vi "CBL Write Block.vi"(4 "TimeOut":u32, 5 "DataNum":u32, 6 "pData":string, 7 "FlashStartAddr":u32, 8 "error in (no error)":errorcluster, 9 "NodeAddr":u8, 10 "CANIndex":i32, 11 "DevIndex":i32) -> (0 "error out":errorcluster, 3 "function return":i32)   [LabVIEW 2012, in "CANBootloader.lvlib"]
doc: "int WINAPI CBL_WriteBlock(int DevIndex,int CANIndex,unsigned char NodeAddr,unsigned int FlashStartAddr,unsigned char *pData,unsigned int DataNum,unsigned int TimeOut);"
uses:
  CANBootloader.lvlib
  Ginkgo_Driver.dll
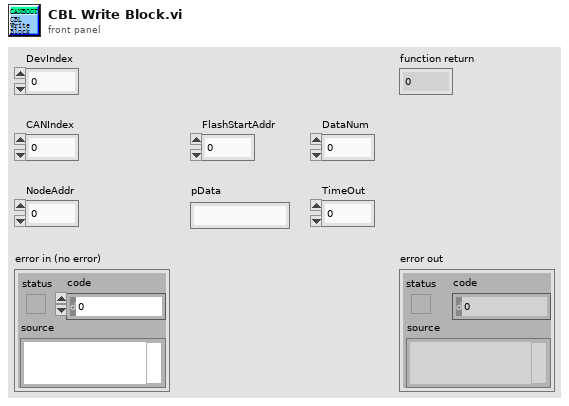
[diagram p1: front panel]
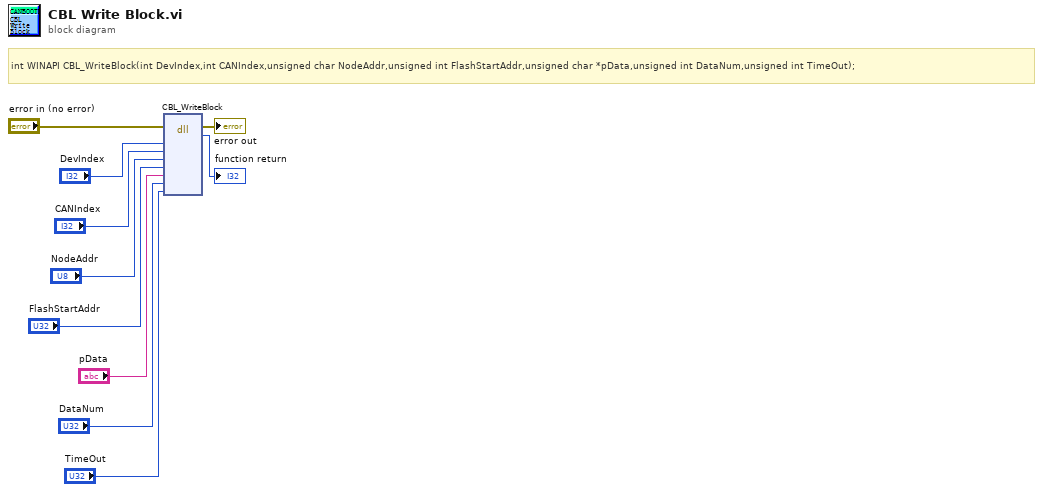
[diagram p0: block diagram]
diagram:
  # "int WINAPI CBL_WriteBlock(int DevIndex,int CANIndex,unsigned char NodeAddr,unsigned int FlashStartAddr,unsigned char *pData,unsigned int DataNum,unsigned int TimeOut);"
  n1 = dll-call lib="E:/Project/vt_ginkgo/truck/Ginkgo Driver/vs2010/Ginkgo_USB-I2C_API_v2.0.3.0/lib/labview_32bit/CANBootloader/Ginkgo_Driver.*" fn="CBL_WriteBlock"(error in="error in (no error)", "DevIndex"="DevIndex", "CANIndex"="CANIndex", "NodeAddr"="NodeAddr", "FlashStartAddr"="FlashStartAddr", "pData"="pData", "DataNum"="DataNum", "TimeOut"="TimeOut") -> (error out=→"error out":errorcluster, →"function return":i32)  [unwired: 9 in, 1 out]
